vi "Progress Bars Open.vi"(7 "Method":enum16{"Open New", "Close", "Get"}(ring)) -> (3 "Open Progress Bars":i16)   [LabVIEW 2016, in "Progress Bar.lvclass"]
doc: "Keeps track of the total number of open progress bars. Functional Global\n\nCopyright: MGI\nAuthored by: Derek Trepanier"
uses:
  <userlib>/_MGI/User Interface/Progress Bar/Progress Bar.lvclass
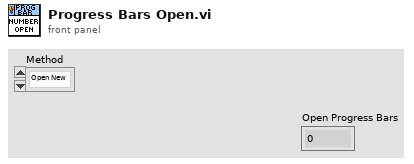
[diagram p1: front panel]
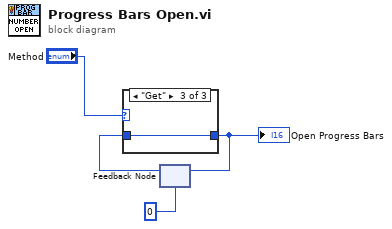
[diagram p0: block diagram]
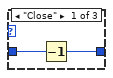
[diagram p2: hidden frame]
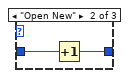
[diagram p3: hidden frame]
diagram:
  n1 = feedback #1(i16 0) -> (w2:i16)
  n2 = case shown="\"Get\"" "Method" {
    tunnel: [w5 w8 w9] -> w3
    tunnel: w2 -> [w6 w7 w9]
    frame "Close" {
      n3 = Decrement(x=w6) -> (x-1=w5:i16)
    }
    frame "Open New" {
      n4 = Increment(x=w7) -> (x+1=w8:i16)
    }
    frame "Get" {
    }
  }
  "Open Progress Bars" <- w3
  n5 = feedback-in #1(w3) -> ()
